vi "UserInput (SubVI).vi"(0 "Display Queue In":refnum<queue>, 5 "Phone number":string, 7 "Parcel number":string, 9 "User Input":string, 11 "Error In":errorcluster, 12 "UserInputState":T1) -> (4 "Display Queue Out":refnum<queue>, 6 "Phone number":string, 8 "Parcel number":string, 10 "UserInputState 2":T1=enum."Withdrawal", 14 "Parcel locker":string, 15 "Error Out":errorcluster)   [LabVIEW 2017]
doc: "Manages the state in which the ATM is operating.s"
uses:
  Controls/DisplayControl.ctl
  Controls/DisplayCommand.ctl
  Controls/UserInputState.ctl
  Controls/MenuItem.ctl
  Controls/AccountsFileCommand.ctl
  Controls/EnableDisableCommand.ctl
  Controls/UpdateMessageControl.ctl
  Controls/UpdateMessageCommand.ctl
  Controls/UpdateMenuCommand.ctl
  Controls/GlobalParcelLocker.vi
  Global 2.vi
panel:
  out "Parcel locker":u32
  out "element":T2
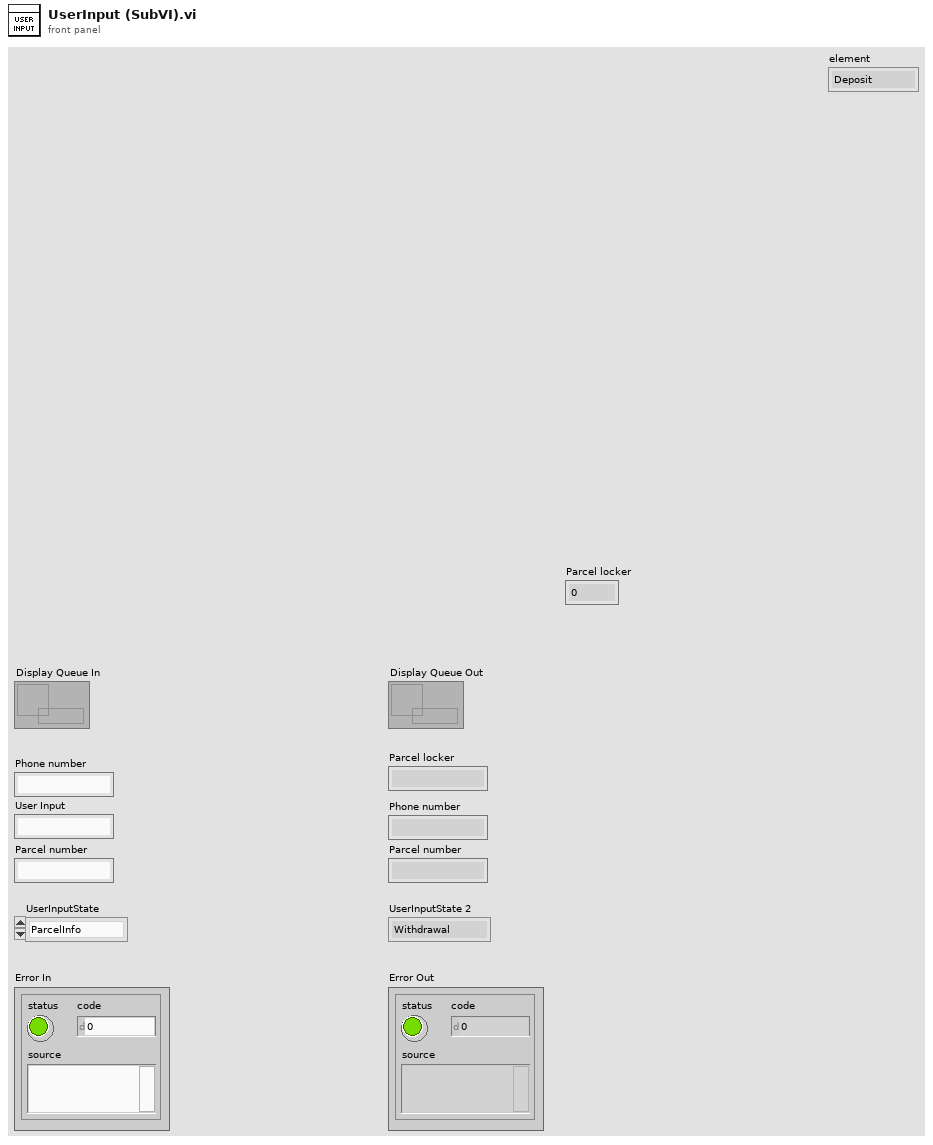
[diagram p1: front panel]
types:
  T1 = typedef "UserInputState.ctl" = enum16{"ParcelInfo", "PhoneInfo", "Deposit", "Withdrawal"}
  T2 = typedef "MenuItem.ctl" = enum16{"Deposit", "Finish", "Withdraw", "None"}
  T3 = typedef "AccountsFileCommand.ctl" = enum16{"Withdrawal", "GetPhoneNumber", "Deposit", "GetParcelNumber"}
  T4 = typedef "DisplayControl.ctl" = cluster{"Command":T5, "Data":variant}
  T5 = typedef "DisplayCommand.ctl" = enum16{"Initialize", "Open/Close Parcel", "Enable/Disable Controls", "FocusCursor", "UpdateMessage", "UpdateMenus", "FinishOperation", "Exit", "CleanUserInput"}
  T6 = typedef "UpdateMenuCommand.ctl" = enum16{"MainMenu", "NoMenu"}
  T7 = typedef "UpdateMessageControl.ctl" = cluster{"Command":T8, "Data":variant}
  T8 = typedef "UpdateMessageCommand.ctl" = enum16{"SystemCrash2", "SystemCrash1", "Welcome", "MainMenu", "PhoneNumberFailed", "PhoneNumberSuccess", "ParcelNumberSuccess", "ParcelNumbertFailed", "SessionTerminate", "SessionFinished", "Deposit", "DepositComplete", "Withdrawal", "WithdrawalComplete", "WithdrawalFailed"}
  T9 = typedef "EnableDisableCommand.ctl" = enum16{"InitialSetup", "StartOperation", "EnableUserInput", "DisableUserInput", "EnableMenus", "DisableMenus"}
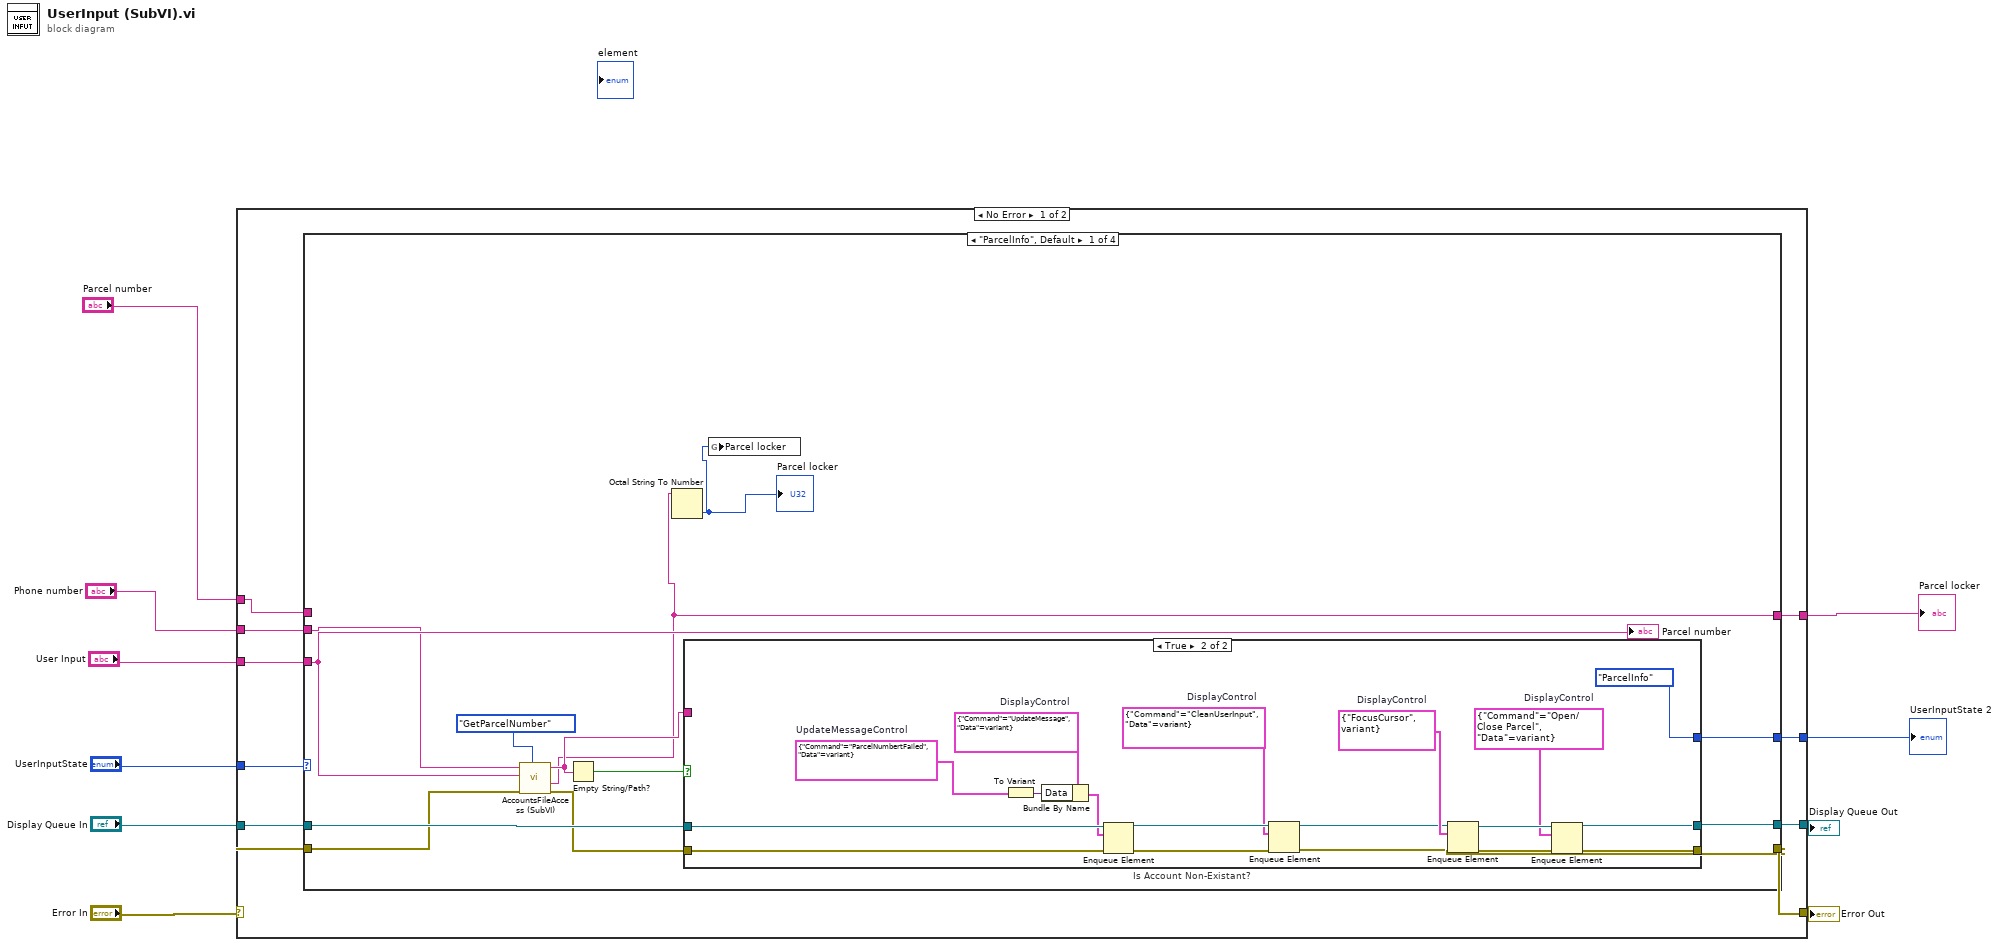
[diagram p0: block diagram]
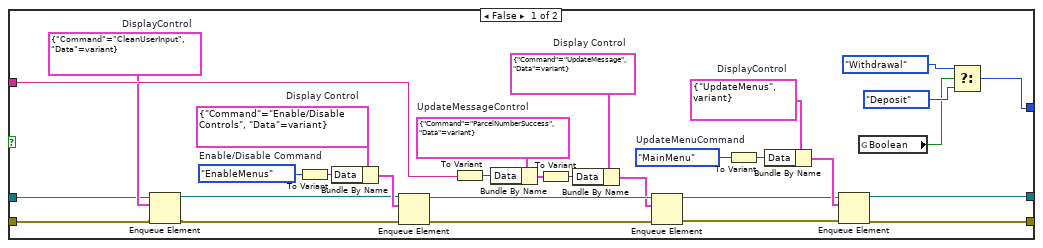
[diagram p2: hidden frame]
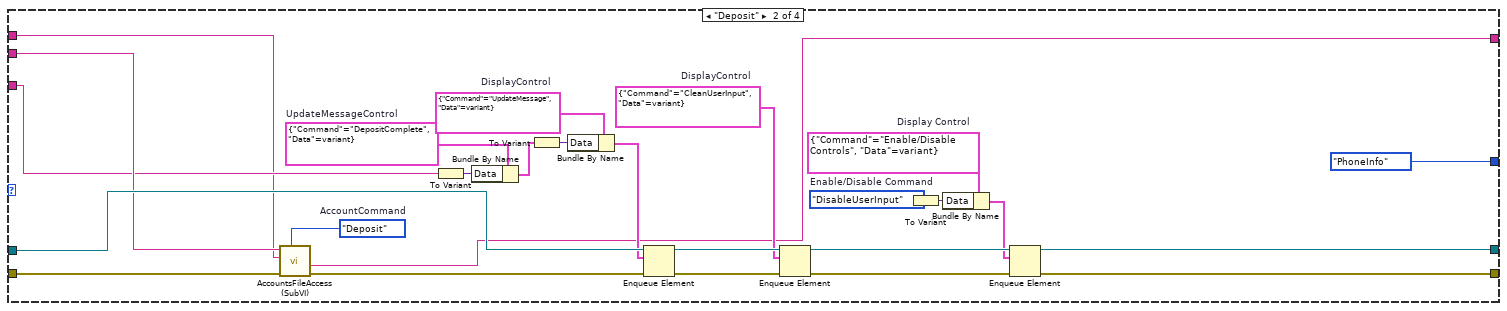
[diagram p3: hidden frame]
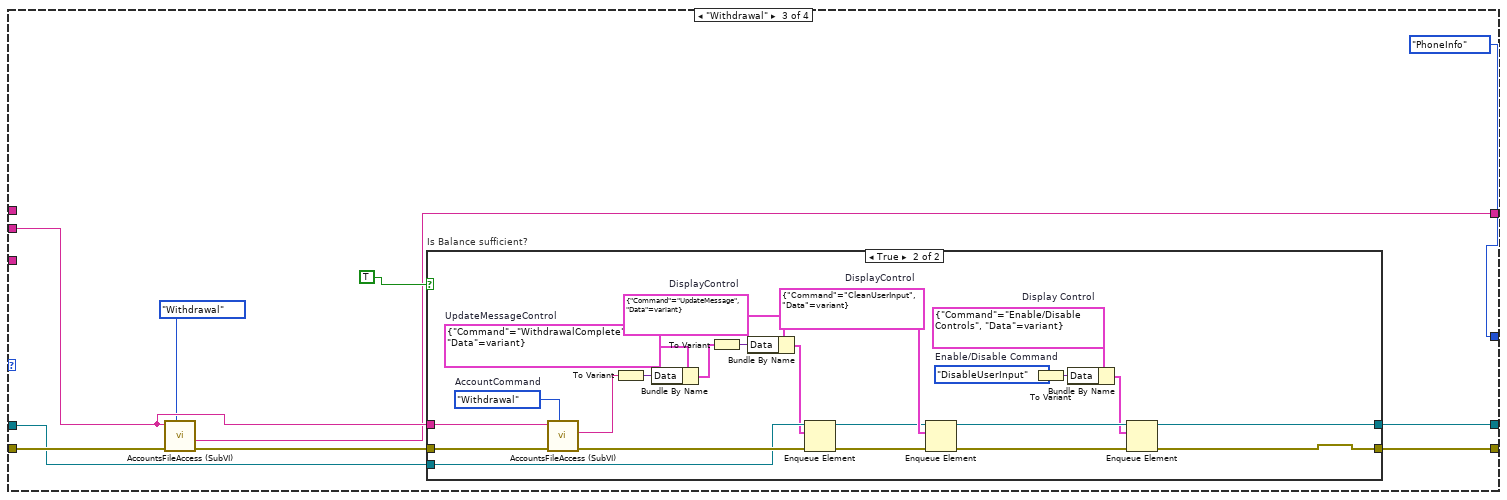
[diagram p4: hidden frame]
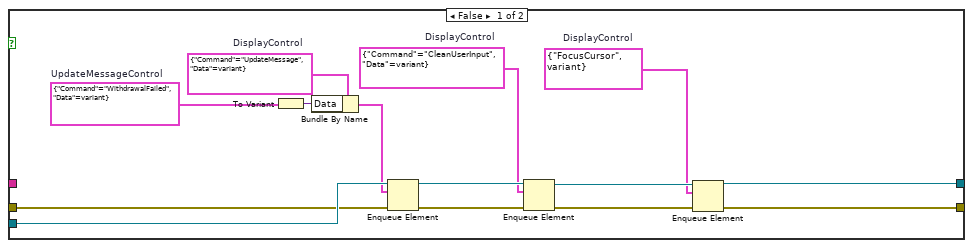
[diagram p5: hidden frame]
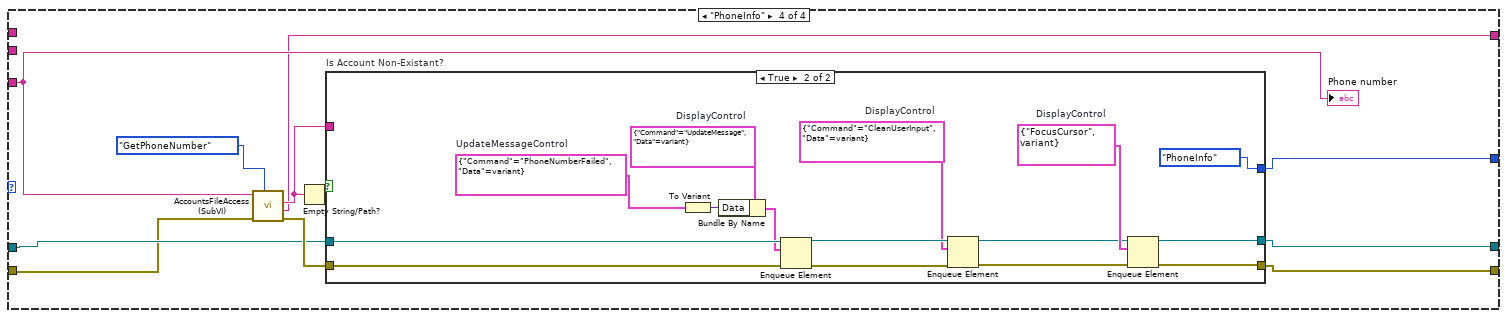
[diagram p6: hidden frame]
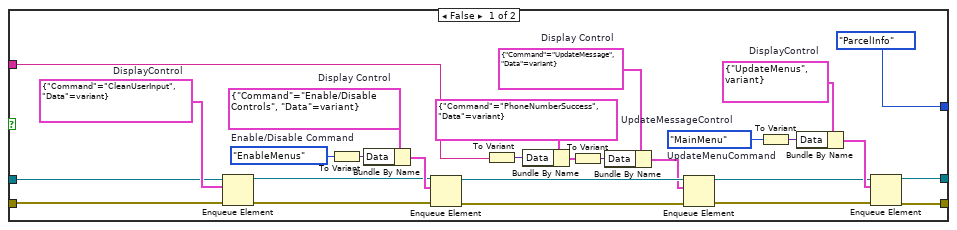
[diagram p7: hidden frame]
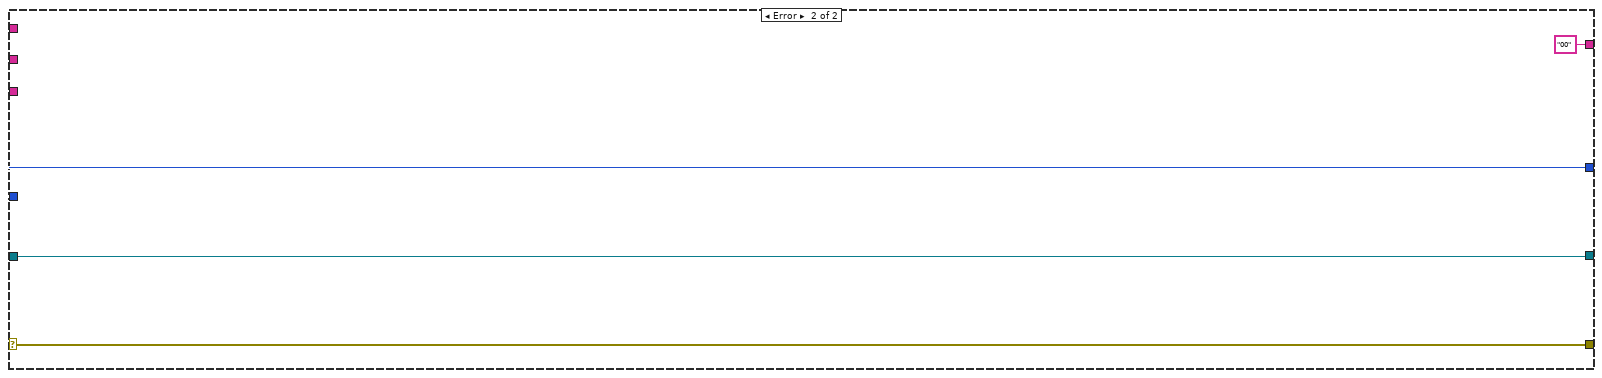
[diagram p8: hidden frame]
diagram:
  n1 = case shown="No Error" "Error In" {
    selector: "Error In" -> [w20 w211]
    tunnel: [w17 w211] -> w9
    tunnel: "Display Queue In" -> [w19 w210]
    tunnel: [w18 w210] -> w7
    tunnel: "User Input" -> [w16 _]
    tunnel: "UserInputState" -> [w15 w209]
    tunnel: "Phone number" -> [w14 _]
    tunnel: "Parcel number" -> [w13 _]
    tunnel: [w12 w209] -> w2
    tunnel: [w11 "00" ("Parcel locker")] -> w1
    frame No Error {
      n2 = case shown="\"ParcelInfo\", Default" w15 {
        tunnel: w19 -> [w32 w104 w115 w161]
        tunnel: w20 -> [w30 w106 w117 w160]
        tunnel: [w27 w89 w114 w159] -> w18
        tunnel: w16 -> [w24 w85 _ w156]
        tunnel: [w28 w90 w113 w158] -> w17
        tunnel: w14 -> [w23 w94 w112 _]
        tunnel: w13 -> [_ w84 _ _]
        tunnel: [w25 UserInputState."PhoneInfo" ("UserInputState 2") UserInputState."PhoneInfo" ("UserInputState 2") w157] -> w12
        tunnel: [w21 w82 w108 w155] -> w11
        frame "ParcelInfo", Default {
          n3 = call "AccountsFileAccess (SubVI).vi"("AccountCommand"=AccountsFileCommand."GetParcelNumber" ("Command"), "Error In"=w30, "Parcel number"=w24, "Phone number"=w23) -> ("Error Out"=w31:errorcluster, "Parcel locker"=w21:string, "Parcel number"=w26:string)  [unwired: 4 in, 1 out]
          n4 = Empty String/Path?(string/path=w26) -> (empty?=w33:bool)
          n5 = Octal String To Number(4:w21) -> (0:w22:u32)  [unwired: 2 in, 1 out]
          "Parcel locker" <- w22
          n6 = case "Is Account Non-Existant?" shown="True" w33 {
            tunnel: w32 -> [w41 w81]
            tunnel: w31 -> [w39 w80]
            tunnel: [w46 w65] -> w27
            tunnel: w26 -> [w51 _]
            tunnel: [w45 w66] -> w28
            tunnel: [w35 UserInputState."ParcelInfo" ("UserInputState 3")] -> w25
            frame False {
              w42 = T4 {"Command"=enum."CleanUserInput", "Data"=variant}  # DisplayControl
              w48 = T4 {"Command"=enum."UpdateMenus", "Data"=variant}  # DisplayControl
              w47 = UpdateMenuCommand."MainMenu"  # UpdateMenuCommand
              w54 = T7 {"Command"=enum."ParcelNumberSuccess", "Data"=variant}  # UpdateMessageControl
              w56 = T4 {"Command"=enum."UpdateMessage", "Data"=variant}  # Display Control
              w60 = EnableDisableCommand."EnableMenus"  # Enable/Disable Command
              w62 = T4 {"Command"=enum."Enable/Disable Controls", "Data"=variant}  # Display Control
              n7 = Enqueue Element(queue=w41, element=w42, error in (no error)=w39) -> (queue out=w40:refnum<queue>, error out=w38:errorcluster)  [unwired: 1 in, 1 out]
              n8 = To Variant(anything=w60) -> (Variant=w63:variant)
              n9 = Bundle By Name(cluster=w62, "Data"=w63) -> (w61:T4)
              n10 = Enqueue Element(queue=w40, element=w61, error in (no error)=w38) -> (queue out=w58:refnum<queue>, error out=w57:errorcluster)  [unwired: 1 in, 1 out]
              n11 = To Variant(anything=w51) -> (Variant=w53:variant)
              n12 = Bundle By Name(cluster=w54, "Data"=w53) -> (w52:T7)
              n13 = To Variant(anything=w52) -> (Variant=w59:variant)
              n14 = Bundle By Name(cluster=w56, "Data"=w59) -> (w55:T4)
              n15 = Enqueue Element(queue=w58, element=w55, error in (no error)=w57) -> (queue out=w44:refnum<queue>, error out=w43:errorcluster)  [unwired: 1 in, 1 out]
              n16 = To Variant(anything=w47) -> (Variant=w50:variant)
              n17 = Bundle By Name(cluster=w48, "Data"=w50) -> (w49:T4)
              n18 = Enqueue Element(queue=w44, element=w49, error in (no error)=w43) -> (queue out=w46:refnum<queue>, error out=w45:errorcluster)  [unwired: 1 in, 1 out]
              n19 = global read "Global 2.vi" "Boolean"() -> (w34:bool)
              n20 = Select(t=UserInputState."Withdrawal" ("UserInputState"), s=w34, f=UserInputState."Deposit" ("UserInputState")) -> (s? t:f=w35:T1)
            }
            frame True {
              w64 = T4 {"Command"=enum."Open/Close Parcel", "Data"=variant}  # DisplayControl
              w70 = T7 {"Command"=enum."ParcelNumbertFailed", "Data"=variant}  # UpdateMessageControl
              w71 = T4 {"Command"=enum."CleanUserInput", "Data"=variant}  # DisplayControl
              w77 = T4 {"Command"=enum."FocusCursor", "Data"=variant}  # DisplayControl
              w79 = T4 {"Command"=enum."UpdateMessage", "Data"=variant}  # DisplayControl
              n21 = To Variant(anything=w70) -> (Variant=w76:variant)
              n22 = Bundle By Name(cluster=w79, "Data"=w76) -> (w78:T4)
              n23 = Enqueue Element(queue=w81, element=w78, error in (no error)=w80) -> (queue out=w72:refnum<queue>, error out=w75:errorcluster)  [unwired: 1 in, 1 out]
              n24 = Enqueue Element(queue=w72, element=w71, error in (no error)=w75) -> (queue out=w73:refnum<queue>, error out=w74:errorcluster)  [unwired: 1 in, 1 out]
              n25 = Enqueue Element(queue=w73, element=w77, error in (no error)=w74) -> (queue out=w68:refnum<queue>, error out=w67:errorcluster)  [unwired: 1 in, 1 out]
              n26 = Enqueue Element(queue=w68, element=w64, error in (no error)=w67) -> (queue out=w65:refnum<queue>, error out=w66:errorcluster)  [unwired: 1 in, 1 out]
            }
          }
          n27 = global write "GlobalParcelLocker.vi" "Parcel locker"(w22) -> ()
          "Parcel number" <- w24
        }
        frame "Deposit" {
          w93 = EnableDisableCommand."DisableUserInput"  # Enable/Disable Command
          w87 = T4 {"Command"=enum."Enable/Disable Controls", "Data"=variant}  # Display Control
          w98 = T4 {"Command"=enum."CleanUserInput", "Data"=variant}  # DisplayControl
          w96 = T7 {"Command"=enum."DepositComplete", "Data"=variant}  # UpdateMessageControl
          w102 = T4 {"Command"=enum."UpdateMessage", "Data"=variant}  # DisplayControl
          w107 = AccountsFileCommand."Deposit"  # AccountCommand
          n28 = call "AccountsFileAccess (SubVI).vi"("AccountCommand"=w107, "Error In"=w106, "Parcel number"=w84, "Phone number"=w94) -> ("Error Out"=w105:errorcluster, "Parcel locker"=w82:string)  [unwired: 4 in, 2 out]
          n29 = To Variant(anything=w85) -> (Variant=w97:variant)
          n30 = Bundle By Name(cluster=w96, "Data"=w97) -> (w95:T7)
          n31 = To Variant(anything=w95) -> (Variant=w103:variant)
          n32 = Bundle By Name(cluster=w102, "Data"=w103) -> (w101:T4)
          n33 = Enqueue Element(queue=w104, element=w101, error in (no error)=w105) -> (queue out=w100:refnum<queue>, error out=w99:errorcluster)  [unwired: 1 in, 1 out]
          n34 = Enqueue Element(queue=w100, element=w98, error in (no error)=w99) -> (queue out=w92:refnum<queue>, error out=w91:errorcluster)  [unwired: 1 in, 1 out]
          n35 = To Variant(anything=w93) -> (Variant=w86:variant)
          n36 = Bundle By Name(cluster=w87, "Data"=w86) -> (w88:T4)
          n37 = Enqueue Element(queue=w92, element=w88, error in (no error)=w91) -> (queue out=w89:refnum<queue>, error out=w90:errorcluster)  [unwired: 1 in, 1 out]
        }
        frame "Withdrawal" {
          n38 = call "AccountsFileAccess (SubVI).vi"("AccountCommand"=AccountsFileCommand."Withdrawal" ("Command"), "Error In"=w117, "Phone number"=w112) -> ("Error Out"=w116:errorcluster, "Parcel locker"=w108:string)  [unwired: 5 in, 2 out]
          n39 = case "Is Balance sufficient?" shown="True" TRUE {
            tunnel: w112 -> [_ w153]
            tunnel: w116 -> [w126 w152]
            tunnel: w115 -> [w127 w143]
            tunnel: [w122 w133] -> w114
            tunnel: [w121 w132] -> w113
            frame False {
              w118 = T4 {"Command"=enum."FocusCursor", "Data"=variant}  # DisplayControl
              w123 = T7 {"Command"=enum."WithdrawalFailed", "Data"=variant}  # UpdateMessageControl
              w125 = T4 {"Command"=enum."CleanUserInput", "Data"=variant}  # DisplayControl
              w130 = T4 {"Command"=enum."UpdateMessage", "Data"=variant}  # DisplayControl
              n40 = To Variant(anything=w123) -> (Variant=w131:variant)
              n41 = Bundle By Name(cluster=w130, "Data"=w131) -> (w124:T4)
              n42 = Enqueue Element(queue=w127, element=w124, error in (no error)=w126) -> (queue out=w129:refnum<queue>, error out=w128:errorcluster)  [unwired: 1 in, 1 out]
              n43 = Enqueue Element(queue=w129, element=w125, error in (no error)=w128) -> (queue out=w120:refnum<queue>, error out=w119:errorcluster)  [unwired: 1 in, 1 out]
              n44 = Enqueue Element(queue=w120, element=w118, error in (no error)=w119) -> (queue out=w122:refnum<queue>, error out=w121:errorcluster)  [unwired: 1 in, 1 out]
            }
            frame True {
              w139 = EnableDisableCommand."DisableUserInput"  # Enable/Disable Command
              w138 = T4 {"Command"=enum."Enable/Disable Controls", "Data"=variant}  # Display Control
              w151 = T4 {"Command"=enum."CleanUserInput", "Data"=variant}  # DisplayControl
              w145 = T7 {"Command"=enum."WithdrawalComplete", "Data"=variant}  # UpdateMessageControl
              w147 = T4 {"Command"=enum."UpdateMessage", "Data"=variant}  # DisplayControl
              w154 = AccountsFileCommand."Withdrawal"  # AccountCommand
              n45 = call "AccountsFileAccess (SubVI).vi"("AccountCommand"=w154, "Error In"=w152, "Phone number"=w153) -> ("Error Out"=w144:errorcluster, "Phone number"=w140:string)  [unwired: 5 in, 2 out]
              n46 = To Variant(anything=w140) -> (Variant=w146:variant)
              n47 = Bundle By Name(cluster=w145, "Data"=w146) -> (w141:T7)
              n48 = To Variant(anything=w141) -> (Variant=w148:variant)
              n49 = Bundle By Name(cluster=w147, "Data"=w148) -> (w142:T4)
              n50 = Enqueue Element(queue=w143, element=w142, error in (no error)=w144) -> (queue out=w149:refnum<queue>, error out=w150:errorcluster)  [unwired: 1 in, 1 out]
              n51 = Enqueue Element(queue=w149, element=w151, error in (no error)=w150) -> (queue out=w137:refnum<queue>, error out=w136:errorcluster)  [unwired: 1 in, 1 out]
              n52 = To Variant(anything=w139) -> (Variant=w134:variant)
              n53 = Bundle By Name(cluster=w138, "Data"=w134) -> (w135:T4)
              n54 = Enqueue Element(queue=w137, element=w135, error in (no error)=w136) -> (queue out=w133:refnum<queue>, error out=w132:errorcluster)  [unwired: 1 in, 1 out]
            }
          }
        }
        frame "PhoneInfo" {
          n55 = call "AccountsFileAccess (SubVI).vi"("AccountCommand"=AccountsFileCommand."GetPhoneNumber" ("Command"), "Error In"=w160, "Phone number"=w156) -> ("Error Out"=w164:errorcluster, "Parcel locker"=w155:string, "Phone number"=w163:string)  [unwired: 5 in, 1 out]
          n56 = Empty String/Path?(string/path=w163) -> (empty?=w165:bool)
          n57 = case "Is Account Non-Existant?" shown="True" w165 {
            tunnel: w161 -> [w169 w207]
            tunnel: w164 -> [w166 w206]
            tunnel: [w175 w201] -> w159
            tunnel: w163 -> [w180 _]
            tunnel: [w174 w200] -> w158
            tunnel: [UserInputState."ParcelInfo" ("UserInputState 2") UserInputState."PhoneInfo" ("UserInputState 2")] -> w157
            frame False {
              w170 = T4 {"Command"=enum."CleanUserInput", "Data"=variant}  # DisplayControl
              w177 = T4 {"Command"=enum."UpdateMenus", "Data"=variant}  # DisplayControl
              w176 = UpdateMenuCommand."MainMenu"  # UpdateMenuCommand
              w183 = T7 {"Command"=enum."PhoneNumberSuccess", "Data"=variant}  # UpdateMessageControl
              w185 = T4 {"Command"=enum."UpdateMessage", "Data"=variant}  # Display Control
              w189 = EnableDisableCommand."EnableMenus"  # Enable/Disable Command
              w191 = T4 {"Command"=enum."Enable/Disable Controls", "Data"=variant}  # Display Control
              n58 = Enqueue Element(queue=w169, element=w170, error in (no error)=w166) -> (queue out=w168:refnum<queue>, error out=w167:errorcluster)  [unwired: 1 in, 1 out]
              n59 = To Variant(anything=w189) -> (Variant=w192:variant)
              n60 = Bundle By Name(cluster=w191, "Data"=w192) -> (w190:T4)
              n61 = Enqueue Element(queue=w168, element=w190, error in (no error)=w167) -> (queue out=w187:refnum<queue>, error out=w186:errorcluster)  [unwired: 1 in, 1 out]
              n62 = To Variant(anything=w180) -> (Variant=w182:variant)
              n63 = Bundle By Name(cluster=w183, "Data"=w182) -> (w181:T7)
              n64 = To Variant(anything=w181) -> (Variant=w188:variant)
              n65 = Bundle By Name(cluster=w185, "Data"=w188) -> (w184:T4)
              n66 = Enqueue Element(queue=w187, element=w184, error in (no error)=w186) -> (queue out=w173:refnum<queue>, error out=w172:errorcluster)  [unwired: 1 in, 1 out]
              n67 = To Variant(anything=w176) -> (Variant=w179:variant)
              n68 = Bundle By Name(cluster=w177, "Data"=w179) -> (w178:T4)
              n69 = Enqueue Element(queue=w173, element=w178, error in (no error)=w172) -> (queue out=w175:refnum<queue>, error out=w174:errorcluster)  [unwired: 1 in, 1 out]
            }
            frame True {
              w194 = T7 {"Command"=enum."PhoneNumberFailed", "Data"=variant}  # UpdateMessageControl
              w195 = T4 {"Command"=enum."CleanUserInput", "Data"=variant}  # DisplayControl
              w203 = T4 {"Command"=enum."FocusCursor", "Data"=variant}  # DisplayControl
              w205 = T4 {"Command"=enum."UpdateMessage", "Data"=variant}  # DisplayControl
              n70 = To Variant(anything=w194) -> (Variant=w202:variant)
              n71 = Bundle By Name(cluster=w205, "Data"=w202) -> (w204:T4)
              n72 = Enqueue Element(queue=w207, element=w204, error in (no error)=w206) -> (queue out=w196:refnum<queue>, error out=w199:errorcluster)  [unwired: 1 in, 1 out]
              n73 = Enqueue Element(queue=w196, element=w195, error in (no error)=w199) -> (queue out=w197:refnum<queue>, error out=w198:errorcluster)  [unwired: 1 in, 1 out]
              n74 = Enqueue Element(queue=w197, element=w203, error in (no error)=w198) -> (queue out=w201:refnum<queue>, error out=w200:errorcluster)  [unwired: 1 in, 1 out]
            }
          }
          "Phone number" <- w156
        }
      }
    }
    frame Error {
    }
  }
  "Error Out" <- w9
  "Display Queue Out" <- w7
  "UserInputState 2" <- w2
  "Parcel locker" <- w1
